vi "PH_SHS_Analysis_Statistician.PC Data Collection.vi"(0 "i ref in":refnum<vi>, 2 "Data":T1 {"State" items=["no info", "off/false/out", "on/true/in", "Failure", "Alarm", "Status 1", "Status 2", "Status 3"]; "Zernicke Coefficients"."2nd Spherical" scale=-2.0..2.0 scale format="%.2f"; "Zernicke Coefficients"."2nd Coma y" scale=-2.0..2.0 scale format="%.2f"; "Zernicke Coefficients"."2nd Coma x" scale=-2.0..2.0 scale format="%.2f"; "Zernicke Coefficients"."2nd Astig 45°" scale=-2.0..2.0 scale format="%.2f"; "Zernicke Coefficients"."2nd Astig 0°" scale=-2.0..2.0 scale format="%.2f"; "Zernicke Coefficients"."Trefoil 30°" scale=-2.0..2.0 scale format="%.2f"; "Zernicke Coefficients"."Trefoil 0°" scale=-2.0..2.0 scale format="%.2f"; "Zernicke Coefficients"."Spherical" scale=-2.0..2.0 scale format="%.2f"; "Zernicke Coefficients"."Coma y" scale=-2.0..2.0 scale format="%.2f"; "Zernicke Coefficients"."Coma x" scale=-2.0..2.0 scale format="%.2f"; "Zernicke Coefficients"."Astig 45°" scale=-2.0..2.0 scale format="%.2f"; "Zernicke Coefficients"."Astig 0°" scale=-2.0..2.0 scale format="%.2f"; "Zernicke Coefficients"."Defocus" scale=-2.0..2.0 scale format="%.2f"; "Zernicke Coefficients"."Tilt y" scale=-2.0..2.0 scale format="%.2f"; "Zernicke Coefficients"."Tilt x" scale=-2.0..2.0 scale format="%.2f"}, 5 "error IO":errorcluster) -> (14 "i ref out":refnum<vi>, 19 "error out":errorcluster)   [LabVIEW 2014, in "PH_SHS_Analysis_Statistician.lvlib"]
uses:
  PH_SHS_Analysis_Statistician.lvlib
  PH_SHS_Analysis/PH_SHS_Analysis.Zernike Dataset.ctl
  PH_StatusHandler/PH_StatusHandler.Status.ctl
  PH_SHS_Analysis/PH_SHS_Analysis.Zernike Coefficients.ctl
  PH_Common/PH_Common.lvlib
  PH_SHS_Analysis/PH_SHS_Analysis.lvlib
  PH_StatusHandler/PH_StatusHandler.lvlib
panel:
  in  "no link":bool
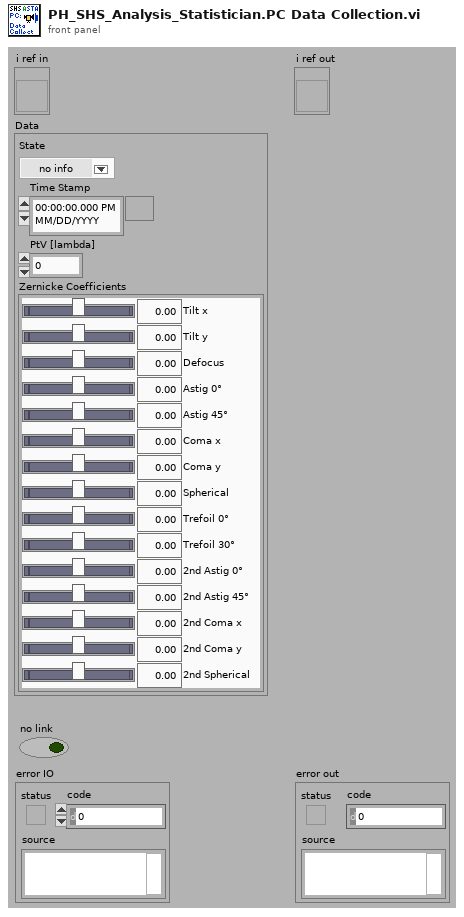
[diagram p1: front panel]
types:
  T1 = typedef "PH_SHS_Analysis.lvlib/PH_SHS_Analysis.Zernike Dataset.ctl" = cluster{"State":T2, "Time Stamp":timestamp, "PtV [lambda]":dbl, "Zernicke Coefficients":T3}
  T2 = typedef "PH_StatusHandler.lvlib/PH_StatusHandler.Status.ctl" = i16
  T3 = typedef "PH_SHS_Analysis.lvlib/PH_SHS_Analysis.Zernike Coefficients.ctl" = cluster{"Tilt x":dbl, "Tilt y":dbl, "Defocus":dbl, "Astig 0°":dbl, "Astig 45°":dbl, "Coma x":dbl, "Coma y":dbl, "Spherical":dbl, "Trefoil 0°":dbl, "Trefoil 30°":dbl, "2nd Astig 0°":dbl, "2nd Astig 45°":dbl, "2nd Coma x":dbl, "2nd Coma y":dbl, "2nd Spherical":dbl}
  T4 = enum8{"Enabled", "Disabled", "Disabled and Grayed Out"}
  T5 = typedef "PH_SHS_Analysis_Statistician.lvlib/PH_SHS_Analysis_Statistician.i attribute.ctl" = cluster{"GUI Refs ":cluster{"Status":refnum<vi>, "Result Graph":refnum<vi>, "Mean Data 1":refnum<vi>, "Std Dev Data 1":refnum<vi>, "Mean Data 2":refnum<vi>, "Std Dev Data 2":refnum<vi>, "Mean Data 3":refnum<vi>, "Std Dev Data 3":refnum<vi>, "Dummy Mean":refnum<vi>, "Dummy Std Dev":refnum<vi>, "Export Data":refnum<vi>, "Data 1":refnum<vi>, "Data 2":refnum<vi>, "Data 3":refnum<vi>, "Stat or Trend":refnum<vi>, "Delete":refnum<vi>, "Analyzer":refnum<vi>, "Current Zernike Coefficients":refnum<vi>, "PtV [Lambda]":refnum<vi>, "sample length":refnum<vi>}, "Analyzer":string, "Stat or Trend":bool, "Data 1":i16, "Data 2":i16, "Data 3":i16, "Data":T1[], "sample length":i32, "Datasets strored":i32, "Dataarray Size":i32}
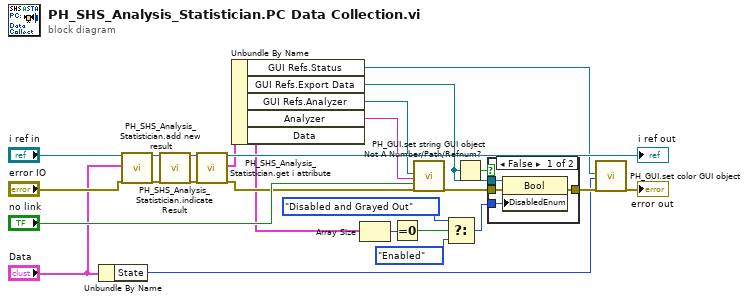
[diagram p0: block diagram]
diagram:
  n1 = Unbundle By Name("Data") -> ("State"=w4:T2)
  n2 = call "PH_SHS_Analysis_Statistician.add new result.vi"("i ref in"="i ref in", "SHS Analyzer Dataset"="Data", "error in (no error)"="error IO") -> ("i ref out"=w2:refnum<vi>, "error out"=w3:errorcluster)  [unwired: 15 in]
  n3 = call "PH_SHS_Analysis_Statistician.indicate Result.vi"("i ref in"=w2, "error in (no error)"=w3) -> ("i ref out"=w10:refnum<vi>, "error out"=w9:errorcluster)  [unwired: 16 in]
  n4 = call "PH_SHS_Analysis_Statistician.get i attribute.vi"("i ref in"=w10, "error in (no error)"=w9) -> ("i ref out"=→"i ref out":refnum<vi>, "i attribute"=w20:T5, "error out"=w8:errorcluster)  [unwired: 15 in]
  n5 = Unbundle By Name(w20) -> ("GUI Refs.Status"=w6:refnum<vi>, "GUI Refs.Export Data"=w14:refnum<vi>, "GUI Refs.Analyzer"=w21:refnum<vi>, "Analyzer"=w19:string, "Data"=w7:T1[])
  n6 = Array Size(array=w7) -> (size(s)=w18:i32)
  n7 = Equal To 0?(x=w18) -> (x = 0?=w17:bool)
  n8 = call "PH_GUI.set string GUI object.vi"("GUI object Ref"=w21, "Text"=w19, "Blinking? (false)"="no link", "error in"=w8) -> ("error out"=w15:errorcluster)  [unwired: 15 in]
  n9 = Select(t=T4."Disabled and Grayed Out", s=w17, f=T4."Enabled" ("Disabled")) -> (s? t:f=w11:T4)
  n10 = Not A Number/Path/Refnum?(number/path/refnum=w14) -> (NaN/Path/Refnum?=w16:bool)
  n11 = case shown="False" w16 {
    tunnel: w15 -> [w30 w31]
    tunnel: [w29 w31] -> w5
    tunnel: w14 -> [w28 _]
    tunnel: w11 -> [w27 _]
    frame False {
      n12 = property class="Bool"(reference=w28, error in=w30, "DisabledEnum"=w27) -> (error out=w29:errorcluster)  [unwired: 1 out]
    }
    frame True {
    }
  }
  n13 = call "PH_GUI.set color GUI object.vi"("GUI object Ref"=w6, "State"=w4, "error in (no error)"=w5) -> ("error out"=→"error out":errorcluster)  [unwired: 16 in]
